vi "Save LCOS Configuration.vi"(11 "LCOS Configuration Ref":refnum<vi>) -> ()   [LabVIEW 2011]
panel:
  out "Error Out":errorcluster
  in  "Error In":errorcluster
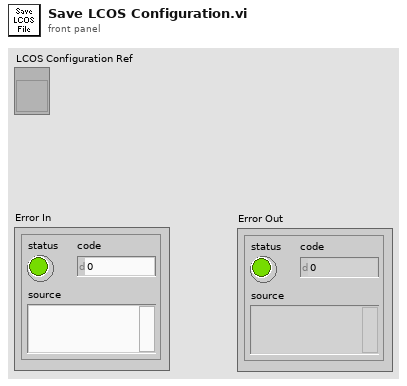
[diagram p1: front panel]
types:
  T1 = cluster{"X pitch":dbl, "rotation":dbl, "Center H":dbl, "Center V":dbl, "# Spots H":u32, "# Spots V":u32, "Spot size":dbl, "ref_spot _dark":bool, "Exact Phase Formula":bool, "phase_wrap_pos":bool, "Set Focus (mm)":dbl, "phase_max":dbl, "phase_factor":u8, "Steer LW":u32, "Steer vmax":u8, "phase_wrap_neg":bool, "steer_horiz":bool, "steer_pad":i64, "steer_only":bool, "Wavelength":dbl, "Y pitch":dbl, "python":bool, "test_pattern":bool, "grid":bool, "dark_all":bool, "Xm_str":string, "Ym_str":string, "ref_spot":i64, "stretch":bool}
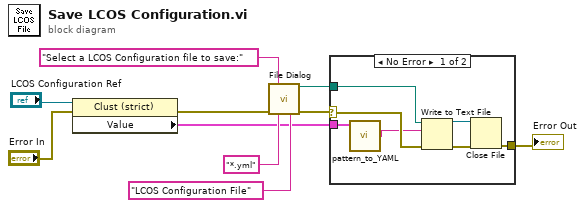
[diagram p0: block diagram]
diagram:
  n1 = property class="Clust (strict)"(reference="LCOS Configuration Ref", error in="Error In") -> (error out=w8:errorcluster, "Value"=w4:T1)  [unwired: 1 out]
  n2 = call "File Dialog"("prompt"="Select a LCOS Configuration file to save:", "error in"=w8, "pattern (all files)"="*.yml", "pattern label"="LCOS Configuration File") -> ("selected path"=w2:path, "error out"=w3:errorcluster)  [unwired: 8 in, 2 out]
  n3 = case shown="No Error" w3 {
    selector: w3 -> [w16 w18]
    tunnel: w4 -> [w17 _]
    tunnel: w2 -> [w14 _]
    tunnel: [w11 w18] -> w1
    frame No Error {
      n4 = call "pattern_to_YAML.vi"("Pattern Definition"=w17) -> ("Result"=w15:string)  [unwired: 3 in]
      n5 = Write to Text File(file (use dialog)=w14, text=w15, error in=w16) -> (refnum out=w12:refnum<file>, error out=w13:errorcluster)  [unwired: 1 in, 1 out]
      n6 = Close File(refnum=w12, error in=w13) -> (error out=w11:errorcluster)  [unwired: 1 out]
    }
    frame Error {
    }
  }
  "Error Out" <- w1
